vi "From Serial Form.vi"(6 "Serial Version":T1, 10 "Deserializer in":refnum<class "Deserializer.lvclass">, 11 "MC Data in":refnum<class "MC Data.lvclass">) -> (0 "error out":errorcluster, 2 "Deserializer out":refnum<class "Deserializer.lvclass">, 3 "MC Data out":refnum<class "MC Data.lvclass">)   [LabVIEW 2014, in "MC Data.lvclass"]
uses:
  MC Data.lvclass
  <vilib>/NI/AQ Character Lineator/Deserializer/Deserializer.lvclass
  <vilib>/NI/AQ Character Lineator/Serialization Common/Serial Version.ctl
  <vilib>/NI/AQ Character Lineator/Serializable/Remove Single.vi
  Alicat Data.lvclass
  <vilib>/NI/AQ Character Lineator/Serializable/Serializable.lvclass
  <vilib>/NI/AQ Character Lineator/Serialization Common/Serialization Common.lvlib
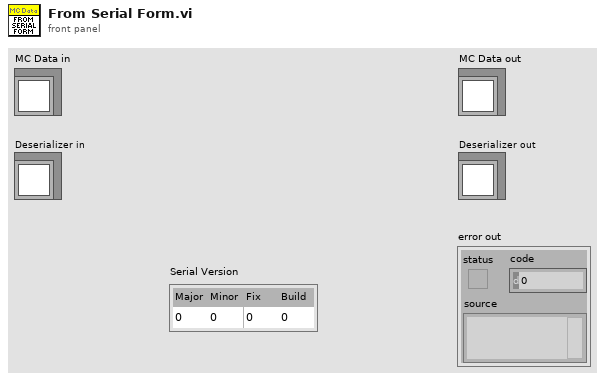
[diagram p1: front panel]
types:
  T1 = typedef "Serialization Common.lvlib/Serial Version.ctl" = cluster{"Major":u16, "Minor":u16, "Fix":u16, "Build":u16}
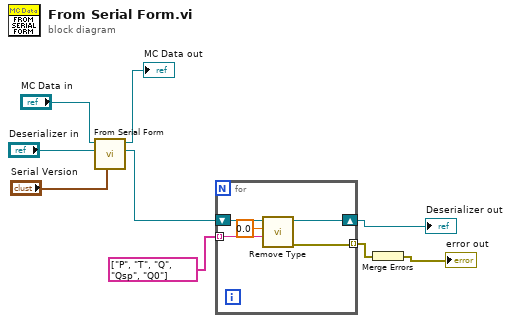
[diagram p0: block diagram]
diagram:
  n1 = call-parent "From Serial Form.vi"("Serial Version"="Serial Version", "Deserializer in"="Deserializer in", "Data in"="MC Data in") -> ("Deserializer out"=w5:refnum<class "Deserializer.lvclass">, "Data out"=→"MC Data out":refnum<class "MC Data.lvclass">)  [unwired: 6 in, 1 out]
  n2 = for {
    shift-right: [w13] -> w3
    shift-left: w5 -> [w14]
    tunnel: string[] ["P", "T", "Q", "Qsp", "Q0"] -> [w12] mode=indexing
    tunnel: [w10] -> w2 mode=indexing
    n3 = call-poly <vilib>:"Remove Type.vi"("Name"=w12, "Default Value"=sgl 0.0, "Deserializer in"=w14) -> ("error out"=w10:errorcluster, "Deserializer out"=w13:refnum<class "Deserializer.lvclass">)  [unwired: 5 in, 2 out]
  }
  "Deserializer out" <- w3
  n4 = Merge Errors(w2) -> (→"error out":errorcluster)
